vi "WIFI下载.vi"(9 "远程端口":u16, 10 "地址":string, 11 "程序":string[](array[string])) -> ()   [LabVIEW 2020]
uses:
  user32.dll
panel:
  out "进度":string
  out "下载进度":i32(slide)
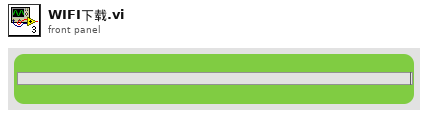
[diagram p1: front panel]
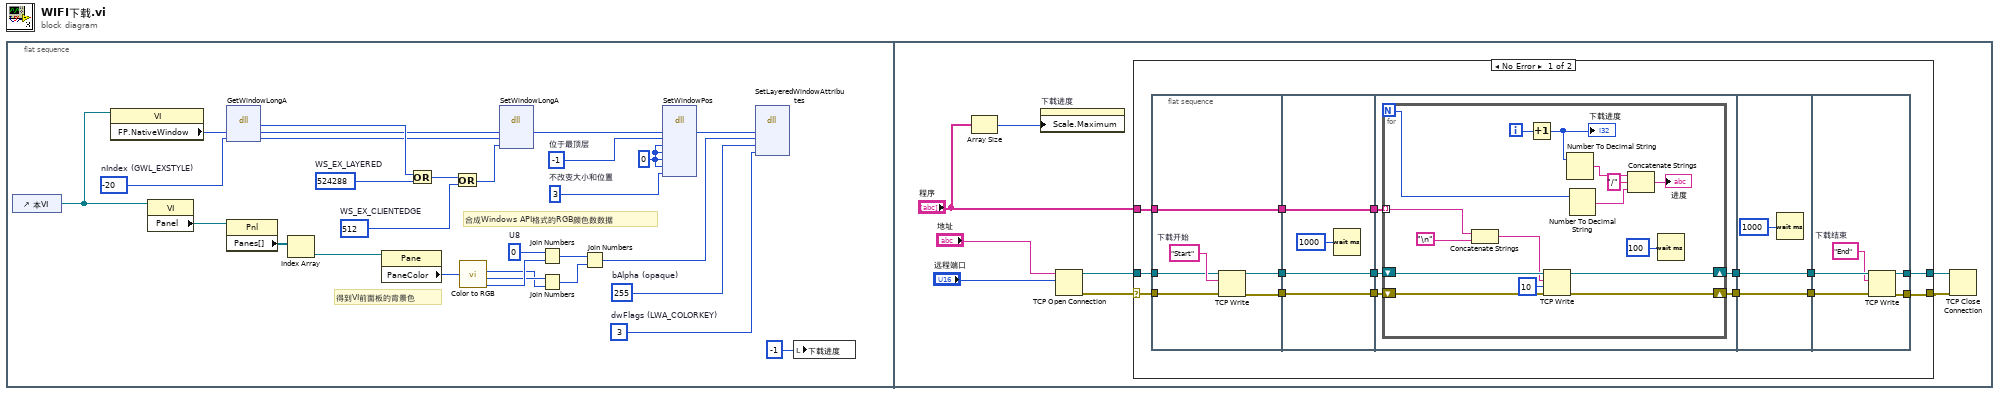
[diagram p0: block diagram]
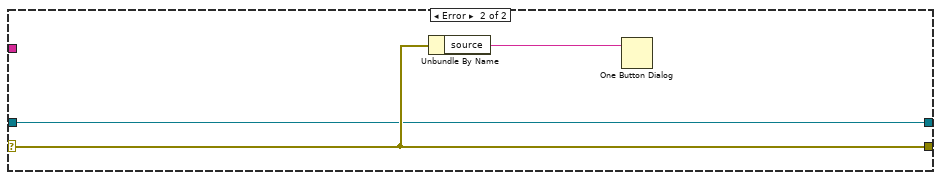
[diagram p2: hidden frame]
diagram:
  n1 = flat-sequence {
    frame #0 {
      w26 = 512  # WS_EX_CLIENTEDGE
      w22 = 3  # 不改变大小和位置
      w25 = 0 ("nIndex")
      w21 = -1  # 位于最顶层
      w3 = 255  # bAlpha (opaque)
      w2 = 3  # dwFlags (LWA_COLORKEY)
      w10 = u8 0  # U8
      w18 = 524288  # WS_EX_LAYERED
      w19 = -20  # nIndex (GWL_EXSTYLE)
      # "合成Windows API格式的RGB颜色数数据"
      # "得到VI前面板的背景色"
      n2 = control-ref of="本VI"() -> (w29:refnum<vi>)
      n3 = property class="VI"(reference=w29) -> ("FP.NativeWindow"=w20:u64)  [unwired: 1 in, 2 out]
      n4 = property class="VI"(reference=w29) -> ("Panel"=w5:refnum<vi>)  [unwired: 1 in, 2 out]
      n5 = dll-call lib="user32.dll" fn="GetWindowLongA"("handle"=w20, "nIndex"=w19) -> ("返回类型"=w17:i32, "handle"=w16:i32, "nIndex"=w15:i32)  [unwired: 3 in, 2 out]
      n6 = property class="Pnl"(reference=w5) -> ("Panes[]"=w6:refnum<vi>[])  [unwired: 1 in, 2 out]
      n7 = Index Array(array=w6) -> (element=w7:refnum<vi>)  [unwired: 1 in]
      n8 = property class="Pane"(reference=w7) -> ("PaneColor"=w11:u32)  [unwired: 1 in, 2 out]
      n9 = Or(x=w17, y=w18) -> (x .or. y?=w27:i32)
      n10 = Or(x=w27, y=w26) -> (x .or. y?=w28:i32)
      n11 = call <vilib>:"Color to RGB.vi"("Color"=w11) -> ("R"=w12:u8, "G"=w13:u8, "B"=w14:u8)  [unwired: 1 out]
      n12 = dll-call lib="USER32.DLL" fn="SetWindowLongA" label="SetWindowLong"("handle"=w16, "nIndex"=w15, "dwNewLong"=w28) -> ("handle"=w23:i32)  [unwired: 5 in, 3 out]
      n13 = Join Numbers(hi=w10, lo=w14) -> ((hi.lo)=w9:u16)
      n14 = Join Numbers(hi=w13, lo=w12) -> ((hi.lo)=w8:u16)
      n15 = Join Numbers(hi=w9, lo=w8) -> ((hi.lo)=w4:u32)
      n16 = dll-call lib="USER32.DLL" fn="SetWindowPos"("hWnd"=w23, "hWndInsertAfter"=w21, "x"=w25, "y"=w25, "cx"=w25, "cy"=w25, "wFlags"=w22) -> ("hWnd"=w24:i32)  [unwired: 9 in, 3 out]
      n17 = dll-call lib="USER32.DLL" fn="SetLayeredWindowAttributes" label="SetLayerdWindowAttributs"("handle"=w24, "crkey"=w4, "bAlpha"=w3, "dwFlags"=w2) -> ()  [unwired: 7 in, 3 out]
      n18 = local write "下载进度"(-1 ("下载中……")) -> ()
    }
    frame #1 {
      n19 = Array Size(array="程序") -> (size(s)=w32:i32)
      n20 = property on="下载进度" class="Slide (strict)"("Scale.Maximum"=w32) -> ()  [unwired: 2 in, 2 out]
      n21 = TCP Open Connection(address="地址", remote port or service name="远程端口") -> (connection ID=w30:refnum<k5>, error out=w33:errorcluster)  [unwired: 3 in]
      n22 = case shown="No Error" w33 {
        selector: w33 -> [w39 w94]
        tunnel: [w46 w92] -> w37
        tunnel: [w47 w94] -> w36
        tunnel: "程序" -> [w52 _]
        tunnel: w30 -> [w38 w92]
        frame No Error {
          n23 = flat-sequence {
            tunnel: w52 -> [w58]
            tunnel: [w53] -> w42
            tunnel: [w58] -> w41
            tunnel: [w54] -> w40
            tunnel: w39 -> [w57]
            tunnel: w38 -> [w55]
            tunnel: [w62] -> w45
            tunnel: [w61] -> w44
            tunnel: [w60] -> w43
            tunnel: w42 -> [w62]
            tunnel: w41 -> [w61]
            tunnel: w40 -> [w60]
            tunnel: [w64] -> w51
            tunnel: [w63] -> w50
            tunnel: w45 -> [w67]
            tunnel: w44 -> [w66]
            tunnel: w43 -> [w65]
            tunnel: w51 -> [w86]
            tunnel: w50 -> [w85]
            tunnel: [w86] -> w49
            tunnel: [w85] -> w48
            tunnel: w49 -> [w90]
            tunnel: w48 -> [w91]
            tunnel: [w89] -> w47
            tunnel: [w88] -> w46
            frame #0 {
              w56 = "Start"  # 下载开始
              n24 = TCP Write(connection ID=w55, data in=w56, error in (no error)=w57) -> (connection ID out=w53:refnum<k5>, error out=w54:errorcluster)  [unwired: 1 in, 1 out]
            }
            frame #1 {
              n25 = Wait (ms)(milliseconds to wait=u32 1000 ("等待时间（毫秒）")) -> ()  [unwired: 1 out]
            }
            frame #2 {
              n26 = for {
                N -> [w69]
                shift-right: [w81] -> w64
                shift-left: w67 -> [w83]
                shift-right: [w80] -> w63
                shift-left: w65 -> [w82]
                tunnel: w66 -> [w79] mode=indexing
                i -> [w70]
                n27 = Concatenate Strings(w79, "\n") -> (w77:string)
                n28 = Increment(x=w70) -> (x+1=w75:i32)
                "下载进度" <- w75
                n29 = TCP Write(connection ID=w83, data in=w77, error in (no error)=w82, 9:10 ("超时毫秒(25000)")) -> (connection ID out=w81:refnum<k5>, error out=w80:errorcluster)  [unwired: 1 out]
                n30 = Number To Decimal String(number=w75) -> (decimal integer string=w74:string)  [unwired: 1 in]
                n31 = Number To Decimal String(number=w69) -> (decimal integer string=w72:string)  [unwired: 1 in]
                n32 = Concatenate Strings(w74, "/" ("字符串"), w72) -> (→"进度":string)
                n33 = Wait (ms)(milliseconds to wait=u32 100 ("等待时间（毫秒）")) -> ()  [unwired: 1 out]
              }
            }
            frame #3 {
              n34 = Wait (ms)(milliseconds to wait=u32 1000 ("等待时间（毫秒）")) -> ()  [unwired: 1 out]
            }
            frame #4 {
              w87 = "End"  # 下载结束
              n35 = TCP Write(connection ID=w90, data in=w87, error in (no error)=w91) -> (connection ID out=w88:refnum<k5>, error out=w89:errorcluster)  [unwired: 1 in, 1 out]
            }
          }
        }
        frame Error {
          n36 = Unbundle By Name(w94) -> ("source"=w93:string)
          n37 = One Button Dialog(message=w93) -> ()  [unwired: 1 in, 1 out]
        }
      }
      n38 = TCP Close Connection(connection ID=w37, error in (no error)=w36) -> ()  [unwired: 1 in, 2 out]
    }
  }
